vi "DCIR_run_1pulse.vi"(6 "3P4S":bool, 7 "Offset%":sgl, 8 "errin":errorcluster, 9 "AmpCharg":dbl, 10 "pathin":path, 11 "VisaAlimIn":refnum<visa-resource-name>) -> (0 "errout":errorcluster, 1 "PV":string, 2 "DATAout":cluster{"Rch":dbl, "A ch":dbl, "max":dbl}, 3 "VisaAlimOut":refnum<visa-resource-name>, 4 "Out":T1, 5 "Cell et DCIR ok":bool)   [LabVIEW 2020]
uses:
  <instrlib>/IT6000C/IT6000C.lvlib
  <userlib>/Alex_Peak_lib/PEAK_lib_ALEX.lvlib
  <userlib>/PCAN Basic/PCANBasic.lvlib
  <userlib>/PCAN Basic/Controls/BaudrateEenum.ctl
  <userlib>/PCAN Basic/Controls/Channel.ctl
  ctrl glo/VG_progressBar.vi
panel:
  out "isPASS?":bool
  out "Rcharge":dbl
  out "Rmax":dbl
  out "V gamme":bool
  in  "stop":bool
  out "Booléen":bool
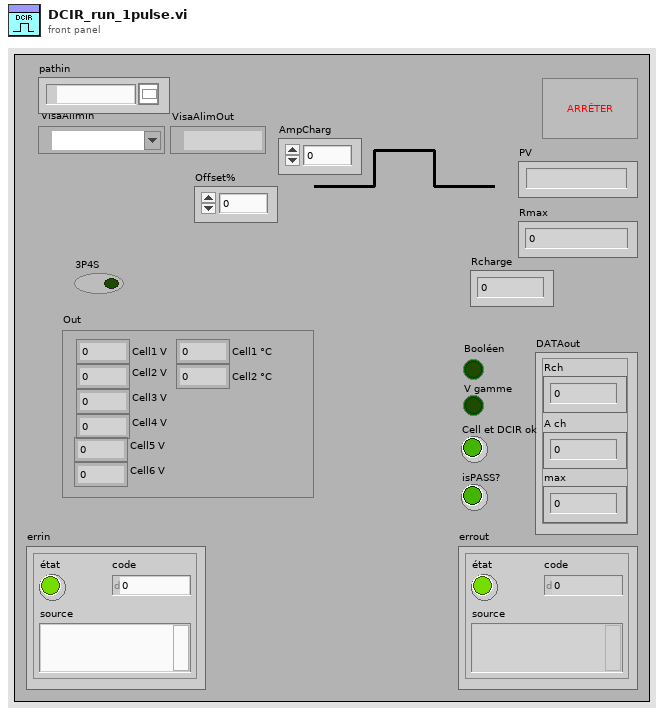
[diagram p1: front panel]
types:
  T1 = cluster{"Cell1 V":sgl, "Cell2 V":sgl, "Cell3 V":sgl, "Cell4 V":sgl, "Cell1 °C":sgl, "Cell2 °C":sgl, "Cell5 V":sgl, "Cell6 V":sgl}
  T2 = typedef "PCANBasic.lvlib/Channel.ctl" = enum16{"PCAN_NONEBUS", "not used1", "not used2", "not used3", "not used4", "not used5", "not used6", "not used7", "not used8", "not used9", "not used10", "not used11", "not used12", "not used13", "not used14", "not used15", "not used16", "not used17", "not used18", "not used19", "not used20", "not used21", "not used22", "not used23", "not used24", "not used25", "not used26", "not used27", "not used28", "not used29", "not used30", "not used31", "not used32", "PCAN_ISABUS1", "PCAN_ISABUS2", "PCAN_ISABUS3", "PCAN_ISABUS4", "PCAN_ISABUS5", "PCAN_ISABUS6", "PCAN_ISABUS7", "PCAN_ISABUS8", "not used41", "not used42", "not used43", "not used44", "not used45", "not used46", "not used47", "not used48", "PCAN_DNGBUS1", "not used50", "not used51", "not used52", "not used53", "not used54", "not used55", "not used56", "not used57", "not used58", "not used59", "not used60", "not used61", "not used62", "not used63", "not used64", "PCAN_PCIBUS1", "PCAN_PCIBUS2", "PCAN_PCIBUS3", "PCAN_PCIBUS4", "PCAN_PCIBUS5", "PCAN_PCIBUS6", "PCAN_PCIBUS7", "PCAN_PCIBUS8", "not used73", "not used74", "not used75", "not used76", "not used77", "not used78", "not used79", "not used80", "PCAN_USBBUS1", "PCAN_USBBUS2", "PCAN_USBBUS3", "PCAN_USBBUS4", "PCAN_USBBUS5", "PCAN_USBBUS6", "PCAN_USBBUS7", "PCAN_USBBUS8", "Not used89", "Not used90", "Not used91", "Not used92", "Not used93", "Not used94", "Not used95", "Not used96", "PCAN_PCCBUS1", "PCAN_PCCBUS2"}
  T3 = typedef "PCANBasic.lvlib/BaudrateEenum.ctl" = enum16{"CAN_Baud_1M", "CAN_Baud_800K", "CAN_BAUD_500K", "CAN_BAUD_250K", "CAN_BAUD_125K", "CAN_BAUD_100K", "CAN_BAUD_95K", "CAN_BAUD_83K", "CAN_BAUD_50K", "CAN_BAUD_47K", "CAN_BAUD_33K", "CAN_BAUD_20K", "CAN_BAUD_10K", "CAN_BAUD_5K", "User Baudrate"}
  T4 = cluster{"Cell1 °C":sgl, "Cell2 °C":sgl, "Cell3 °C":sgl, "Cell4 °C":sgl, "Cell_1_Volt":sgl, "Cell_2_Volt":sgl, "Cell_3_Volt":sgl, "Cell_4_Volt":sgl}
  T5 = cluster{"TempMin":sgl, "TempMax":sgl, "VoltageMin":sgl, "VoltageMax":sgl, "DeltaV":sgl, "DeltaC":sgl, "Ton":sgl}
  T6 = cluster{"ID":u32, "MSGTYPE":u8, "LEN":u8, "DATA[0]":u8, "DATA[1]":u8, "DATA[2]":u8, "DATA[3]":u8, "DATA[4]":u8, "DATA[5]":u8, "DATA[6]":u8, "DATA[7]":u8}
  T7 = cluster{"Cell_1_Temperature":sgl, "Cell_1_Voltage":sgl, "Cell_2_Temperature":sgl, "Cell_2_Voltage":sgl}
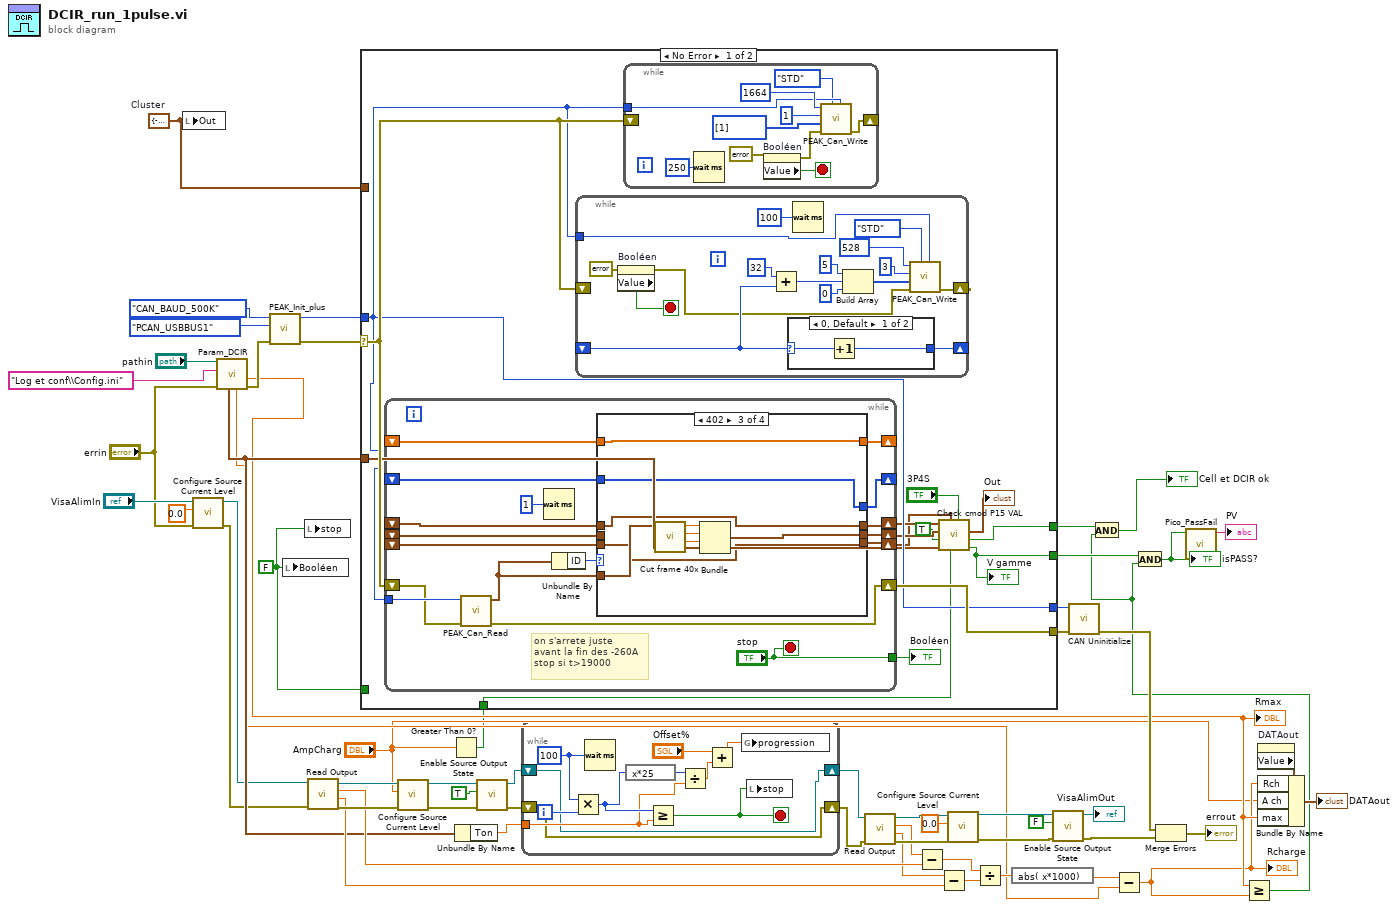
[diagram p0: block diagram]
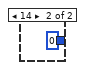
[diagram p2: hidden frame]
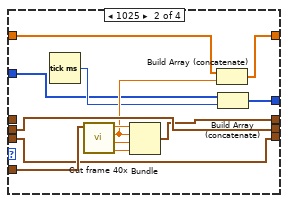
[diagram p4: hidden frame]
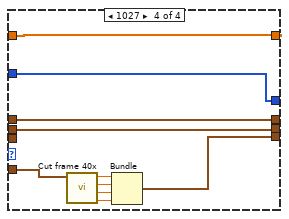
[diagram p5: hidden frame]
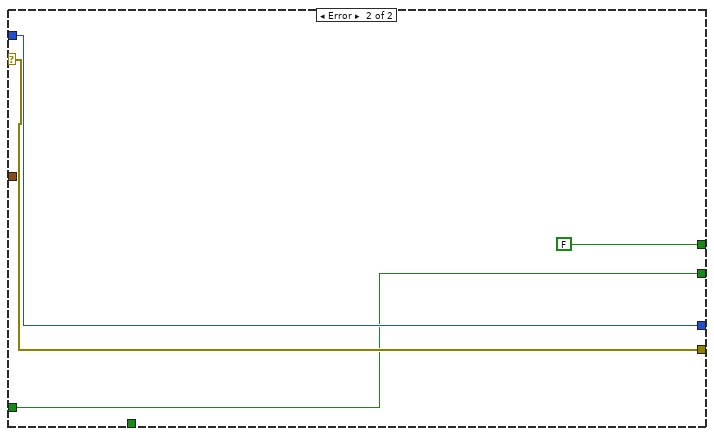
[diagram p6: hidden frame]
diagram:
  w48 = FALSE ("Booléen")
  w3 = T4 {"Cell1 °C"=-1.0, "Cell2 °C"=-1.0, "Cell3 °C"=-1.0, "Cell4 °C"=-1.0, "Cell_1_Volt"=-1.0, "Cell_2_Volt"=-1.0, "Cell_3_Volt"=-1.0, "Cell_4_Volt"=-1.0}  # Cluster
  n1 = local write "Out"(w3) -> ()
  n2 = call <instrlib>:"Configure Source Current Level.vi"("error in (no error)"="errin", "Value(0)"=0.0, "VISA resource name"="VisaAlimIn") -> ("error out"=w12:errorcluster, "VISA resource name out"=w13:refnum<visa-resource-name>)  [unwired: 7 in]
  n3 = call "Param_DCIR.vi"("errin"="errin", "Chaîne"="Log et conf\\Config.ini", "pathin"="pathin") -> ("errout"=w47:errorcluster, "Rmax"=w17:dbl, "Roffset"=w11:dbl, "Data out"=w18:T5)  [unwired: 2 in, 3 out]
  "Rmax" <- w17
  n4 = call <userlib>:"PEAK_Init_plus.vi"("errin"=w47, "Channel"=Channel."PCAN_USBBUS1", "BTR0BTR1"=BaudrateEenum."CAN_BAUD_500K") -> ("errout"=w46:errorcluster, "Channel out"=w45:T2)  [unwired: 7 in]
  n5 = local write "Booléen"(w48) -> ()
  n6 = local write "stop"(w48) -> ()
  n7 = call <instrlib>:"Read Output.vi"("error in (no error)"=w12, "VISA resource name"=w13) -> ("error out"=w43:errorcluster, "Actual Current Level (A)"=w26:dbl, "Actual Voltage Level (V)"=w28:dbl, "VISA resource name out"=w42:refnum<visa-resource-name>)  [unwired: 6 in]
  n8 = call <instrlib>:"Configure Source Current Level.vi"("error in (no error)"=w43, "Value(0)"="AmpCharg", "VISA resource name"=w42) -> ("error out"=w40:errorcluster, "VISA resource name out"=w39:refnum<visa-resource-name>)  [unwired: 7 in]
  n9 = Greater Than 0?(x="AmpCharg") -> (x > 0?=w1:bool)
  n10 = case shown="No Error" w46 {
    selector: w46 -> [w72 w160]
    tunnel: w45 -> [w70 w159]
    tunnel: [w71 w160] -> w53
    tunnel: [w70 w159] -> w54
    tunnel: w18 -> [w68 _]
    tunnel: w48 -> [_ w158]
    tunnel: [w64 w158] -> w21
    tunnel: [w63 FALSE ("ok global")] -> w6
    tunnel: w3 -> [_ _]
    tunnel: w1 -> [w59 _]
    frame No Error {
      n11 = while {
        shift-right: [w111] -> w71
        shift-left: w72 -> [w116]
        shift-right: [w109] -> w67
        shift-left: _ -> [w113]
        shift-right: [w110] -> w66
        shift-left: _ -> [w112]
        tunnel: w70 -> [w117]
        tunnel: ["stop"] -> w69
        shift-right: [w106] -> _
        shift-left: _ -> [w107]
        shift-right: [w104] -> _
        shift-left: _ -> [w105]
        shift-right: [w103] -> w62
        shift-left: _ -> [w102]
        stop <- "stop" stop-if-true
        # "on s'arrete juste \navant la fin des -260A\nstop si t>19000"
        n12 = call <userlib>:"PEAK_Can_Read.vi"("errin"=w116, "Channel out"=w117) -> ("errout"=w111:errorcluster, "MessageBuffer out"=w115:T6)  [unwired: 7 in, 1 out]
        n13 = Wait (ms)(milliseconds to wait=u32 1 ("attente (ms)")) -> ()  [unwired: 1 out]
        n14 = Unbundle By Name(w115) -> ("ID"=w114:u32)
        n15 = case shown="402" w114 {
          tunnel: w115 -> [_ w133 w141 w152]
          tunnel: [w123 w131 w140 w151] -> w109
          tunnel: [w122 w132 w142 w148] -> w110
          tunnel: w113 -> [w123 _ w140 w151]
          tunnel: w112 -> [w122 w132 _ w148]
          tunnel: w107 -> [w121 w130 w139 w150]
          tunnel: [w121 w129 w139 w150] -> w106
          tunnel: w105 -> [w120 w126 w138 w149]
          tunnel: [w120 w125 w138 w149] -> w104
          tunnel: [w119 w124 w137 w147] -> w103
          tunnel: w102 -> [w119 w124 w137 _]
          frame 0, Default {
          }
          frame 1025 {
            n16 = Tick Count (ms)() -> (millisecond timer value=w127:u32)
            n17 = call "Cut frame 40x.vi"("MessageBuffer out"=w133) -> ("Cell_2_Voltage"=w134:sgl, "Cell_2_Temperature"=w135:sgl, "Cell_1_Voltage"=w128:sgl, "Cell_1_Temperature"=w136:sgl)  [unwired: 7 in]
            n18 = Bundle("Cell_1_Temperature"=w136, "Cell_1_Voltage"=w128, "Cell_2_Temperature"=w135, "Cell_2_Voltage"=w134) -> (w131:T7)  [unwired: 1 in]
            n19 = Build Array (concatenate)(w130, w128) -> (w129:sgl[])
            n20 = Build Array (concatenate)(w126, w127) -> (w125:u32[])
          }
          frame 1026 {
            n21 = call "Cut frame 40x.vi"("MessageBuffer out"=w141) -> ("Cell_2_Voltage"=w143:sgl, "Cell_2_Temperature"=w144:sgl, "Cell_1_Voltage"=w145:sgl, "Cell_1_Temperature"=w146:sgl)  [unwired: 7 in]
            n22 = Bundle("Cell_1_Temperature"=w146, "Cell_1_Voltage"=w145, "Cell_2_Temperature"=w144, "Cell_2_Voltage"=w143) -> (w142:T7)  [unwired: 1 in]
          }
          frame 1027 {
            n23 = call "Cut frame 40x.vi"("MessageBuffer out"=w152) -> ("Cell_2_Voltage"=w153:sgl, "Cell_2_Temperature"=w154:sgl, "Cell_1_Voltage"=w155:sgl, "Cell_1_Temperature"=w156:sgl)  [unwired: 7 in]
            n24 = Bundle("Cell_1_Temperature"=w156, "Cell_1_Voltage"=w155, "Cell_2_Temperature"=w154, "Cell_2_Voltage"=w153) -> (w147:T7)  [unwired: 1 in]
          }
        }
      }
      "Booléen" <- w69
      n25 = while {
        tunnel: w70 -> [w83]
        shift-right: [w98] -> _
        shift-left: _ -> [w97]
        shift-right: [w96] -> _
        shift-left: w72 -> [_]
        stop <- w94 stop-if-true
        n26 = property on="Booléen" class="Bool (strict)"(error in=errorcluster {"status"=FALSE, "code"=0, "source"=""} ("entrée d'erreur (pas d'erreur)")) -> (error out=w95:errorcluster, "Value"=w94:bool)  [unwired: 1 in, 1 out]
        n27 = Add(x=u8 32, y=w97) -> (x+y=w89:i32)
        n28 = case shown="0, Default" w97 {
          selector: w97 -> [w100 _]
          tunnel: [w99 0] -> w98
          frame 0, Default {
            n29 = Increment(x=w100) -> (x+1=w99:i32)
          }
          frame 14 {
          }
        }
        n30 = Wait (ms)(milliseconds to wait=u32 100 ("attente (ms)")) -> ()  [unwired: 1 out]
        n31 = Build Array(u8 5 ("élément"), w89, u8 0 ("élément")) -> (w88:i32[])
        n32 = call <userlib>:"PEAK_Can_Write.vi"("CAN Handle"=w83, "MSG type"=enum8{"STD", "RTR", "XTD", "XTD RTR", "STATUS"}."STD", "errin"=w95, "CAN Data"=w88, "DLC (8)"=u8 3, "Identifier"=u32 528) -> ("errout"=w96:errorcluster)  [unwired: 5 in]
      }
      n33 = while {
        tunnel: w70 -> [w75]
        shift-right: [w79] -> _
        shift-left: w72 -> [_]
        stop <- w82 stop-if-true
        n34 = Wait (ms)(milliseconds to wait=u32 250 ("attente (ms)")) -> ()  [unwired: 1 out]
        n35 = property on="Booléen" class="Bool (strict)"(error in=errorcluster {"status"=FALSE, "code"=0, "source"=""} ("entrée d'erreur (pas d'erreur)")) -> (error out=w78:errorcluster, "Value"=w82:bool)  [unwired: 1 in, 1 out]
        n36 = call <userlib>:"PEAK_Can_Write.vi"("CAN Handle"=w75, "MSG type"=enum8{"STD", "RTR", "XTD", "XTD RTR", "STATUS"}."STD", "errin"=w78, "CAN Data"=u8[] [1], "DLC (8)"=u8 1, "Identifier"=u32 1664) -> ("errout"=w79:errorcluster)  [unwired: 5 in]
      }
      n37 = call "Check cmod P15 VAL.vi"("3P4S"="3P4S", "isPos?"=w59, "Cell 5 et 6"=w62, "PostDCIR?"=w68, "intra?"=TRUE, "Cell 3 et 4"=w66, "Cell 1 et 2"=w67) -> ("V gamme"=w64:bool, "ok global"=w63:bool, "Out"=→"Out":T1)  [unwired: 2 out]
      "V gamme" <- w64
    }
    frame Error {
    }
  }
  n38 = Unbundle By Name(w18) -> ("Ton"=w15:sgl)
  n39 = call <instrlib>:"Enable Source Output State.vi"("error in (no error)"=w40, "Enable(True)"=TRUE, "VISA resource name"=w39) -> ("error out"=w10:errorcluster, "VISA resource name out"=w8:refnum<visa-resource-name>)  [unwired: 7 in]
  n40 = while {
    tunnel: w15 -> [w166]
    shift-right: [w164] -> w7
    shift-left: w8 -> [w164]
    shift-right: [w165] -> w9
    shift-left: w10 -> [w165]
    i -> [w171]
    stop <- w169 stop-if-true
    w170 = u32 100 ("attente (ms)")
    n41 = Multiply(x=w170, y=w171) -> (x*y=w167:u32)
    n42 = Wait (ms)(milliseconds to wait=w170) -> ()  [unwired: 1 out]
    n43 = expression code="x*25"(w167) -> (w168:u32)
    n44 = Greater Or Equal?(x=w167, y=w166) -> (x >= y?=w169:bool)
    n45 = Divide(x=w168, y=w166) -> (x/y=w163:sgl)
    n46 = Add(x="Offset%", y=w163) -> (x+y=w161:sgl)
    n47 = global write "VG_progressBar.vi" "progression"(w161) -> ()
    n48 = local write "stop"(w169) -> ()
  }
  n49 = call <instrlib>:"Read Output.vi"("error in (no error)"=w9, "VISA resource name"=w7) -> ("error out"=w37:errorcluster, "Actual Current Level (A)"=w27:dbl, "Actual Voltage Level (V)"=w29:dbl, "VISA resource name out"=w36:refnum<visa-resource-name>)  [unwired: 6 in]
  n50 = Subtract(x=w29, y=w28) -> (x-y=w14:dbl)
  n51 = Subtract(x=w27, y=w26) -> (x-y=w32:dbl)
  n52 = call <instrlib>:"Configure Source Current Level.vi"("error in (no error)"=w37, "Value(0)"=0.0, "VISA resource name"=w36) -> ("error out"=w35:errorcluster, "VISA resource name out"=w34:refnum<visa-resource-name>)  [unwired: 7 in]
  n53 = Divide(x=w14, y=w32) -> (x/y=w31:dbl)
  n54 = expression code="abs( x*1000)"(w31) -> (w30:dbl)
  n55 = call <instrlib>:"Enable Source Output State.vi"("error in (no error)"=w35, "Enable(True)"=FALSE, "VISA resource name"=w34) -> ("error out"=w25:errorcluster, "VISA resource name out"=→"VisaAlimOut":refnum<visa-resource-name>)  [unwired: 7 in]
  n56 = call <userlib>:"CAN Uninitialize.vi"("error in (no error)"=w53, "Channel"=w54) -> ("error out"=w49:errorcluster)  [unwired: 7 in, 2 out]
  n57 = Subtract(x=w30, y=w11) -> (x-y=w16:dbl)
  "Rcharge" <- w16
  n58 = Merge Errors(w49, w25) -> (→"errout":errorcluster)
  n59 = Greater Or Equal?(x=w17, y=w16) -> (x >= y?=w5:bool)
  n60 = And(x=w6, y=w5) -> (x .and. y?=→"Cell et DCIR ok":bool)
  n61 = And(x=w21, y=w5) -> (x .and. y?=w20:bool)
  "isPASS?" <- w20
  n62 = call "Pico_PassFail.vi"("Booléen"=w20) -> ("Vout"=→"PV":string)  [unwired: 10 in]
  n63 = property on="DATAout" class="Clust (strict)"() -> ("Value"=w56:cluster{"Rch":dbl, "A ch":dbl, "max":dbl})  [unwired: 2 in, 2 out]
  n64 = Bundle By Name(cluster=w56, "Rch"=w16, "A ch"="AmpCharg", "max"=w17) -> (→"DATAout":cluster{"Rch":dbl, "A ch":dbl, "max":dbl})
